vi "PLL data source -- meta.vi"(6 "set-get delay (msec)":i64, 7 "data source action":T1=enum."get", 9 "z  in (V)":cdb, 10 "Freq in (Hz)":dbl=40000.0 format="%#_13g") -> (1 "z out (V)":cdb=0.00010527635459-2.9308681405e-05i, 2 "Freq out (Hz)":dbl=55115.2)   [LabVIEW 2018]
uses:
  data source action.ctl
  publisher action.ctl
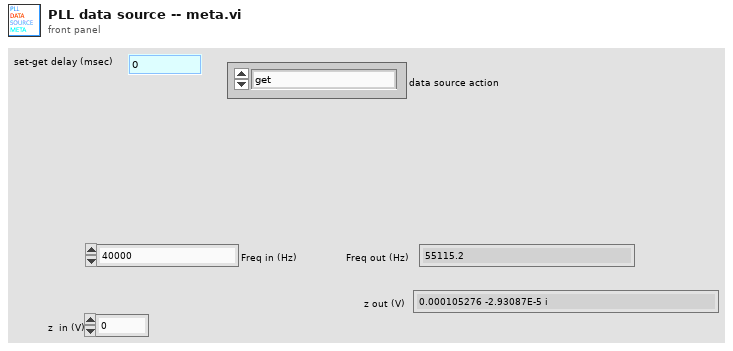
[diagram p1: front panel]
types:
  T1 = typedef "data source action.ctl" = enum16{"set", "get", "init", "set-and-get"}
  T2 = typedef "publisher action.ctl" = enum16{"set", "get", "init", "check"}
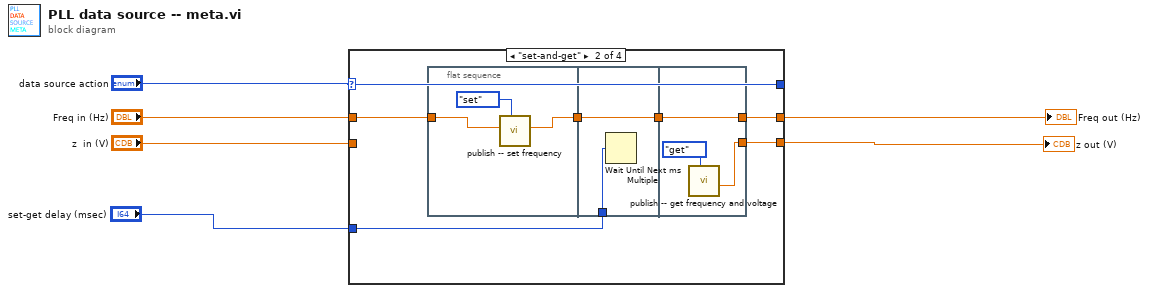
[diagram p0: block diagram]
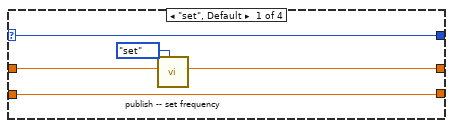
[diagram p2: hidden frame]
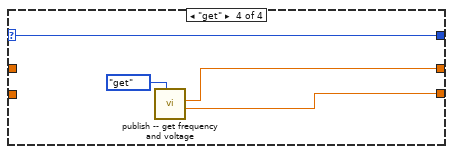
[diagram p4: hidden frame]
diagram:
  n1 = case shown="\"set-and-get\"" "data source action" {
    selector: "data source action" -> [w8 w16 w28 w31]
    tunnel: [w9 w17 w29 w32] -> w5
    tunnel: "Freq in (Hz)" -> [w10 w18 w29 _]
    tunnel: [w8 w16 w28 w31] -> _
    tunnel: "set-get delay (msec)" -> [_ w13 _ _]
    tunnel: [w7 w12 w27 w30] -> w1
    tunnel: "z  in (V)" -> [w7 _ w27 _]
    frame "set", Default {
      n2 = call "publish -- set frequency.vi"("publisher action"=publisher_action."set", "freq IN (Hz)"=w10) -> ("freq out (Hz)"=w9:dbl)  [unwired: 9 in]
    }
    frame "set-and-get" {
      n3 = flat-sequence {
        tunnel: w18 -> [w20]
        tunnel: [w19] -> w15
        tunnel: w15 -> [w23]
        tunnel: [w23] -> w14
        tunnel: w13 -> [w22]
        tunnel: [w26] -> w17
        tunnel: w14 -> [w26]
        tunnel: [w24] -> w12
        frame #0 {
          n4 = call "publish -- set frequency.vi"("publisher action"=publisher_action."set", "freq IN (Hz)"=w20) -> ("freq out (Hz)"=w19:dbl)  [unwired: 9 in]
        }
        frame #1 {
          n5 = Wait Until Next ms Multiple(millisecond multiple=w22) -> ()  [unwired: 1 out]
        }
        frame #2 {
          n6 = call "publish -- get frequency and voltage.vi"("publisher action"=publisher_action."get") -> ("Voltage out (V)"=w24:cdb)  [unwired: 8 in, 2 out]
        }
      }
    }
    frame "init" {
    }
    frame "get" {
      n7 = call "publish -- get frequency and voltage.vi"("publisher action"=publisher_action."get") -> ("Voltage out (V)"=w30:cdb, "freq out (Hz)"=w32:dbl)  [unwired: 8 in, 1 out]
    }
  }
  "Freq out (Hz)" <- w5
  "z out (V)" <- w1
